vi "Remove Sensor.vi"(8 "error in (no error)":errorcluster, 11 "Sensor Model in":refnum<class "Sensor Model.lvclass">) -> (0 "error out":errorcluster, 3 "Sensor Model out":refnum<class "Sensor Model.lvclass">)   [LabVIEW 2013, in "Sensor Model.lvlib" / "Sensor Model.lvclass"]
uses:
  Sensor Model.lvclass
  Sensor Model.lvclass/Sensor Model.ctl
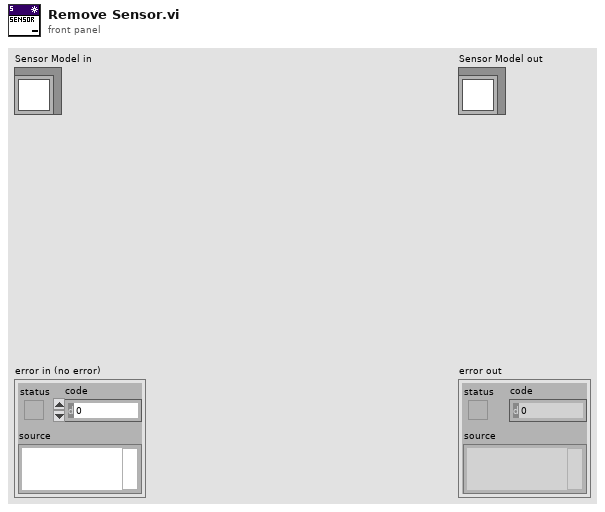
[diagram p1: front panel]
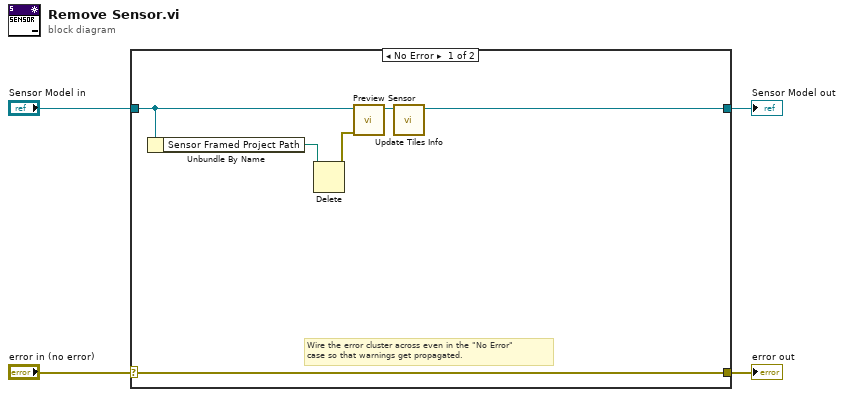
[diagram p0: block diagram]
diagram:
  n1 = case shown="No Error" "error in (no error)" {
    selector: "error in (no error)" -> [w10 w12]
    tunnel: [w10 w12] -> w3
    tunnel: [w7 w11] -> w1
    tunnel: "Sensor Model in" -> [w9 w11]
    frame No Error {
      # "Wire the error cluster across even in the \"No Error\"\ncase so that warnings get propagated."
      n2 = Unbundle By Name(w9) -> ("Sensor Framed Project Path"=w6:path)
      n3 = Delete(path (use dialog)=w6) -> (error out=w5:errorcluster)  [unwired: 4 in, 2 out]
      n4 = call "Preview Sensor.vi"("error in (no error)"=w5, "Sensor Model in"=w9) -> ("Sensor Model out"=w8:refnum<class "Sensor Model.lvclass">)  [unwired: 8 in, 1 out]
      n5 = call "Update Tiles Info.vi"("Sensor Model in"=w8) -> ("Sensor Model out"=w7:refnum<class "Sensor Model.lvclass">)  [unwired: 9 in, 1 out]
    }
    frame Error {
    }
  }
  "error out" <- w3
  "Sensor Model out" <- w1
